vi "FPGA Braking.vi"() -> ()   [LabVIEW 2013]
uses:
  <vilib>/eio/EIONode/EIONode.xnode
  <vilib>/rvi/eio/common/nirviEmuTemplateMethod_errors.vi
panel:
  in  "Boolean":bool
  in  "Cluster":T1
  in  "Enable":bool
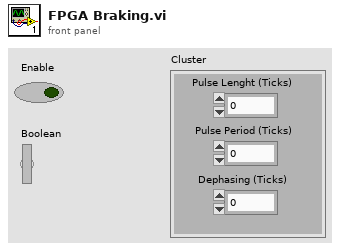
[diagram p1: front panel]
types:
  T1 = cluster{"Pulse Lenght (Ticks)":i16, "Pulse Period (Ticks)":i16, "Dephasing (Ticks)":i16}
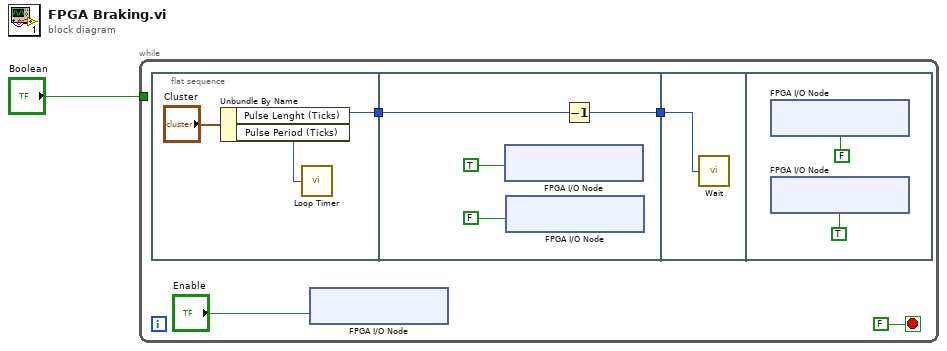
[diagram p0: block diagram]
diagram:
  n1 = while {
    tunnel: "Boolean" -> [_]
    stop <- FALSE stop-if-true
    n2 = flat-sequence {
      tunnel: [w6] -> w2
      tunnel: [w11] -> w5
      tunnel: w2 -> [w9]
      tunnel: w5 -> [w13]
      frame #0 {
        n3 = Unbundle By Name("Cluster") -> ("Pulse Lenght (Ticks)"=w6:i16, "Pulse Period (Ticks)"=w7:i16)
        n4 = call "Loop Timer"("Count(Ticks)"=w7) -> ()  [unwired: 1 out]
      }
      frame #1 {
        n5 = xnode "FPGA I/O Node"("ConnectorC/DIO3"=TRUE ("ConnectorC/DIO7")) -> ()  [unwired: 1 in, 1 out]
        n6 = xnode "FPGA I/O Node"("ConnectorC/DIO7"=FALSE) -> ()  [unwired: 1 in, 1 out]
        n7 = Decrement(x=w9) -> (x-1=w11:i16)
      }
      frame #2 {
        n8 = call "Wait"("Count(Ticks)"=w13) -> ()  [unwired: 1 out]
      }
      frame #3 {
        n9 = xnode "FPGA I/O Node"("ConnectorC/DIO3"=FALSE ("ConnectorC/DIO7")) -> ()  [unwired: 1 in, 1 out]
        n10 = xnode "FPGA I/O Node"("ConnectorC/DIO7"=TRUE) -> ()  [unwired: 1 in, 1 out]
      }
    }
    n11 = xnode "FPGA I/O Node"("ConnectorA/DIO0"="Enable") -> ()  [unwired: 1 in, 1 out]
  }
